vi "CFWSWebClient.vi"(4 "Scan Period":dbl format="%.2f", 5 "Previous Scan Value":dbl format="%.2f", 6 "Present scan array":dbl[](array[numeric]) format="%.2f", 7 "Value to Output":dbl format="%.2f", 8 "Ch Description":T1={"Ch Name"="", "Type"="", "Function"=enum."Analogue Input", "Ch State"=enum."On", "Calibration type"="", "A"=0.0, "B"=0.0, "C"=0.0, "D"=0.0, "Comments"="", "Address"={"Main"=0, "Ch."=0, "Sub"=0, "Port Name"=""}, "String"="", "Duty"=65535} {"Duty" format="%016b"; "D" format="%#_5g"; "C" format="%#_5g"; "B" format="%#_5g"; "A" format="%#_5g"}, 9 "Ch names":string[](array[string])) -> (0 "Scan comment":string, 1 "Output":dbl format="%.3f")   [LabVIEW 2016]
uses:
  ADAM Client/Sub VIs/ADAM Controls/Ch_description_ADAM.ctl
  ADAM Client/Sub VIs/ADAM Controls/Module_type_ADAM.ctl
  ADAM Client/Sub VIs/ADAM Controls/Function_ADAM.ctl
  ADAM Client/Sub VIs/ADAM Controls/Channel_State.ctl
  ADAM Client/Sub VIs/ADAM Controls/Calib_type_ADAM.ctl
  ADAM Client/Sub VIs/ADAM Controls/Address.ctl
  ADAM Client/Sub VIs/ADAM Controls/Remember_value_mode.ctl
panel:
  out "TimeToUpdate?":bool
  in  "stop":bool
  out "Time Of Value (s)":dbl format="%.2f"
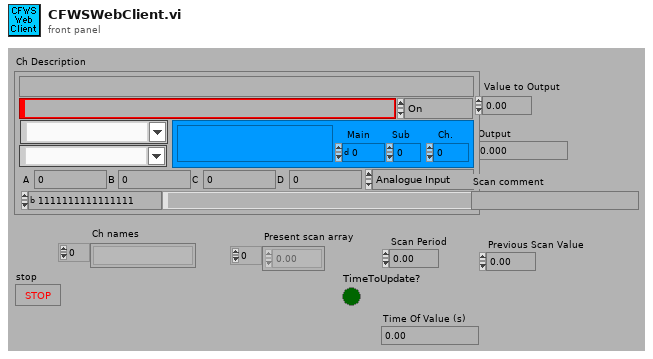
[diagram p1: front panel]
types:
  T1 = typedef "Ch_description_ADAM.ctl" = cluster{"Ch Name":string, "Type":T2, "Function":T3, "Ch State":T4, "Calibration type":T5, "A":dbl, "B":dbl, "C":dbl, "D":dbl, "Comments":string, "Address":T6, "String":string, "Duty":u16}
  T2 = typedef "Module_type_ADAM.ctl" = string
  T3 = typedef "Function_ADAM.ctl" = enum16{"Analogue Input", "Digital Input", "Event counter", "Event rate", "Analogue Output", "Digital Output", "Relay Output"}
  T4 = typedef "Channel_State.ctl" = enum16{"On", "Off", "Always On", "Always Off"}
  T5 = typedef "Calib_type_ADAM.ctl" = string
  T6 = typedef "Address.ctl" = cluster{"Main":i32, "Ch.":i32, "Sub":i32, "Port Name":string}
  T7 = typedef "Remember_value_mode.ctl" = enum16{"Read only", "Read and Write"}
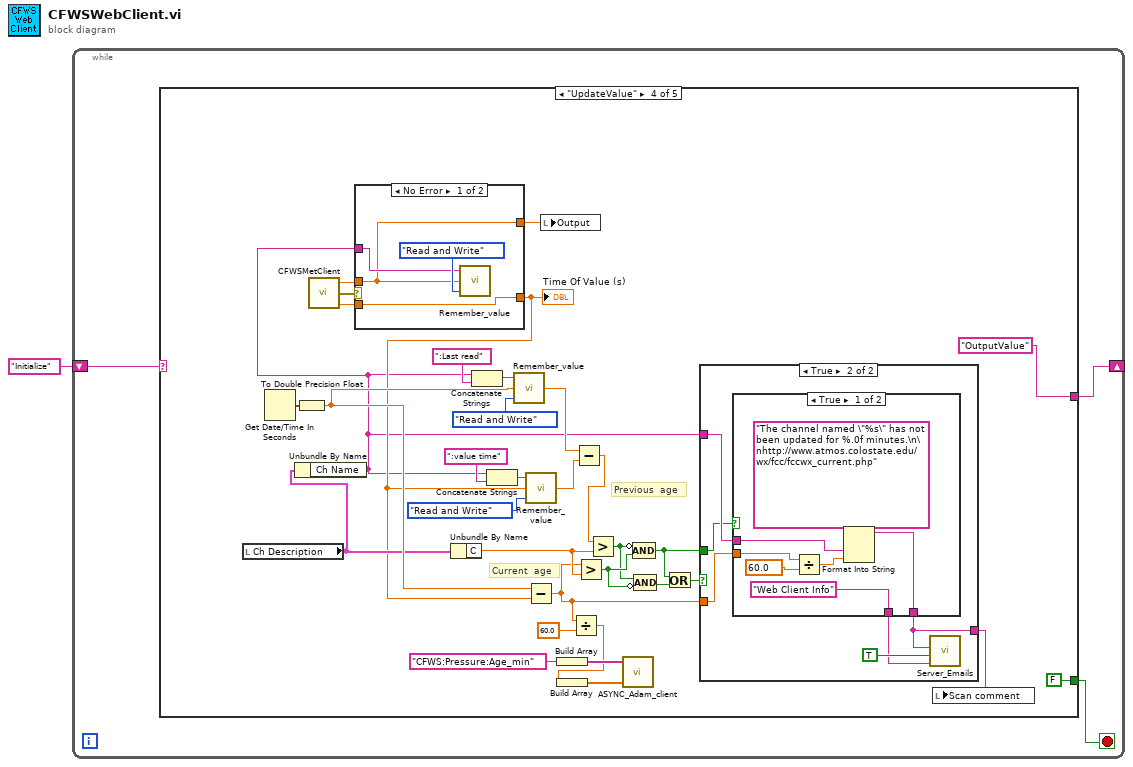
[diagram p0: block diagram]
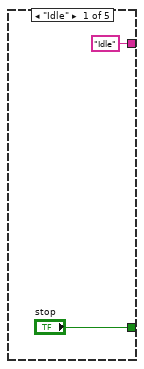
[diagram p2: hidden frame]
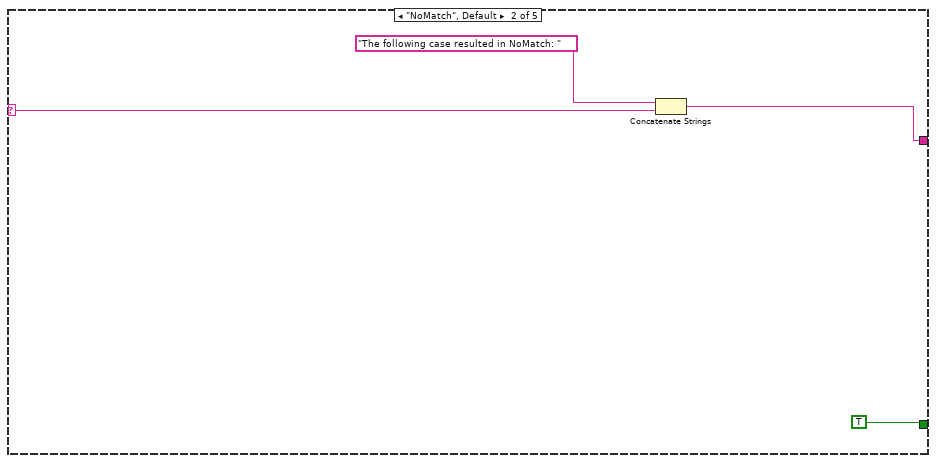
[diagram p3: hidden frame]
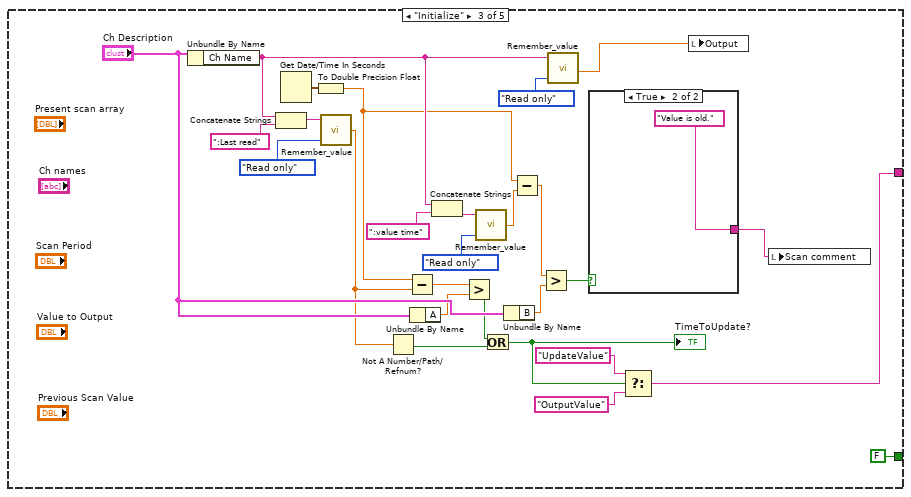
[diagram p4: hidden frame]
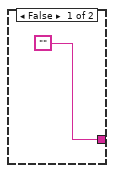
[diagram p5: hidden frame]
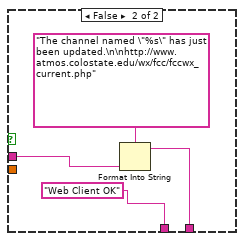
[diagram p7: hidden frame]
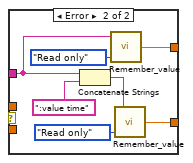
[diagram p8: hidden frame]
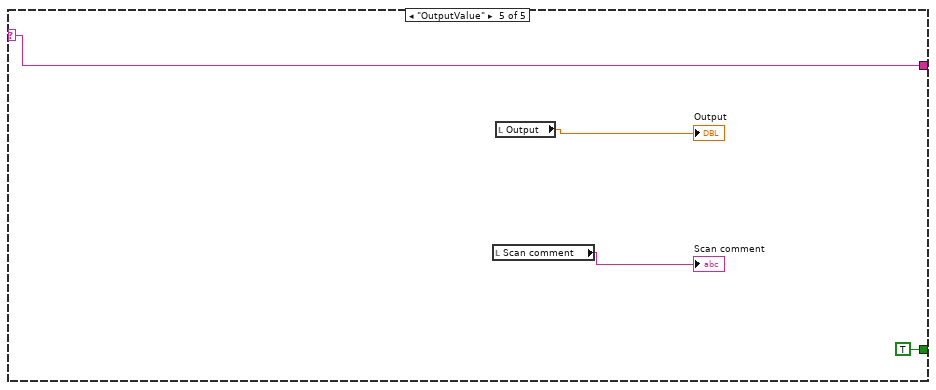
[diagram p9: hidden frame]
diagram:
  n1 = while {
    shift-right: [w3] -> _
    shift-left: "Initialize" -> [w4]
    stop <- w2 stop-if-true
    n2 = case shown="\"UpdateValue\"" w4 {
      selector: w4 -> [_ w8 _ _ w105]
      tunnel: ["Idle" w7 w11 "OutputValue" w105] -> w3
      tunnel: ["stop" TRUE FALSE ("stop") FALSE ("stop") TRUE ("stop")] -> w2
      frame "Idle" {
      }
      frame "NoMatch", Default {
        n3 = Concatenate Strings("The following case resulted in NoMatch: " ("string"), w8) -> (w7:string)
      }
      frame "Initialize" {
        n4 = Unbundle By Name("Ch Description") -> ("Ch Name"=w33:string)
        n5 = Concatenate Strings(w33, ":Last read" ("Substring")) -> (w20:string)
        n6 = Get Date/Time In Seconds() -> (seconds since 1Jan1904=w25:timestamp)
        n7 = To Double Precision Float(number=w25) -> (double precision float=w27:dbl)
        n8 = call "Remember_value.vi"("Mode"=Remember_value_mode."Read only", "Ch name"=w20) -> ("Output Value"=w21:dbl)  [unwired: 1 in]
        n9 = Not A Number/Path/Refnum?(number/path/refnum=w21) -> (NaN/Path/Refnum?=w23:bool)
        n10 = Subtract(x=w27, y=w21) -> (x-y=w17:dbl)
        n11 = Unbundle By Name("Ch Description") -> ("A"=w34:dbl)
        n12 = Concatenate Strings(w33, ":value time" ("Substring")) -> (w31:string)
        n13 = Greater?(x=w17, y=w34) -> (0:w22:bool)
        n14 = call "Remember_value.vi"("Mode"=Remember_value_mode."Read only", "Ch name"=w31) -> ("Output Value"=w26:dbl)  [unwired: 1 in]
        n15 = Or(x=w22, y=w23) -> (x .or. y?=w14:bool)
        "TimeToUpdate?" <- w14
        n16 = Unbundle By Name("Ch Description") -> ("B"=w35:dbl)
        n17 = Subtract(x=w27, y=w26) -> (x-y=w28:dbl)
        n18 = Greater?(x=w28, y=w35) -> (0:w24:bool)
        n19 = call "Remember_value.vi"("Mode"=Remember_value_mode."Read only", "Ch name"=w33) -> ("Output Value"=w16:dbl)  [unwired: 1 in]
        n20 = case shown="True" w24 {
          tunnel: ["" "Value is old." ("Format String")] -> w15
          frame False {
          }
          frame True {
          }
        }
        n21 = Select(t="UpdateValue", s=w14, f="OutputValue") -> (s? t:f=w11:string)
        n22 = local write "Output"(w16) -> ()
        n23 = local write "Scan comment"(w15) -> ()
      }
      frame "UpdateValue" {
        # "Previous  age"
        # "Current  age"
        n24 = local read "Ch Description"() -> (w54:T1)
        n25 = Get Date/Time In Seconds() -> (seconds since 1Jan1904=w63:timestamp)
        n26 = Unbundle By Name(w54) -> ("Ch Name"=w52:string)
        n27 = To Double Precision Float(number=w63) -> (double precision float=w69:dbl)
        n28 = call "CFWSMetClient.vi"() -> ("Time Of Value (s)"=w42:dbl, "error out"=w41:errorcluster, "RawPressure/mBar"=w40:dbl)
        n29 = case shown="No Error" w41 {
          tunnel: [w91 w95] -> w72
          tunnel: [w94 w96] -> w53
          tunnel: w52 -> [w92 w98]
          tunnel: w40 -> [w91 _]
          tunnel: w42 -> [w94 _]
          frame No Error {
            n30 = call "Remember_value.vi"("Mode"=Remember_value_mode."Read and Write", "Input Value"=w91, "Ch name"=w92) -> ()  [unwired: 1 out]
          }
          frame Error {
            n31 = Concatenate Strings(w98, ":value time" ("Substring")) -> (w97:string)
            n32 = call "Remember_value.vi"("Mode"=Remember_value_mode."Read only", "Ch name"=w98) -> ("Output Value"=w95:dbl)  [unwired: 1 in]
            n33 = call "Remember_value.vi"("Mode"=Remember_value_mode."Read only", "Ch name"=w97) -> ("Output Value"=w96:dbl)  [unwired: 1 in]
          }
        }
        "Time Of Value (s)" <- w53
        n34 = Unbundle By Name(w54) -> ("C"=w71:dbl)
        n35 = Concatenate Strings(w52, ":Last read" ("Substring")) -> (w68:string)
        n36 = Concatenate Strings(w52, ":value time" ("Substring")) -> (w57:string)
        n37 = call "Remember_value.vi"("Mode"=Remember_value_mode."Read and Write", "Input Value"=w69, "Ch name"=w68) -> ("Output Value"=w70:dbl)
        n38 = call "Remember_value.vi"("Mode"=Remember_value_mode."Read and Write", "Input Value"=w53, "Ch name"=w57) -> ("Output Value"=w64:dbl)
        n39 = Subtract(x=w69, y=w53) -> (x-y=w45:dbl)
        n40 = local write "Output"(w72) -> ()
        n41 = Build Array("CFWS:Pressure:Age_min") -> (w46:string[])
        n42 = Divide(x=w45, y=60.0) -> (x/y=w43:dbl)
        n43 = Build Array(w43) -> (w47:dbl[])
        n44 = Subtract(x=w70, y=w64) -> (x-y=w65:dbl)
        n45 = Greater?(x=w45, y=w71) -> (0:w59:bool)
        n46 = Greater?(x=w65, y=w71) -> (0:w58:bool)
        n47 = call "ASYNC_Adam_client.vi"("Values"=w47, "Channel Names"=w46) -> ()  [unwired: 1 in, 2 out]
        n48 = Compound Arithmetic op=AND(invert w58, w59) -> (w62:bool)
        n49 = Compound Arithmetic op=AND(w58, invert w59) -> (w60:bool)
        n50 = Or(x=w62, y=w60) -> (x .or. y?=w61:bool)
        n51 = case shown="True" w61 {
          tunnel: w45 -> [_ w79]
          tunnel: w52 -> [_ w78]
          tunnel: w62 -> [_ w77]
          tunnel: ["" w74] -> w51
          frame False {
          }
          frame True {
            n52 = case shown="True" w77 {
              tunnel: w79 -> [w84 _]
              tunnel: w78 -> [w86 w90]
              tunnel: [w81 w88] -> w74
              tunnel: ["Web Client Info" ("Subject") "Web Client OK" ("Subject")] -> w75
              frame True {
                n53 = Divide(x=w84, y=60.0) -> (x/y=w83:dbl)
                n54 = Format Into String(format string="The channel named \"%s\" has not been updated for %.0f minutes.\n\nhttp://www.atmos.colostate.edu/wx/fcc/fccwx_current.php" ("Format String"), w86, w83) -> (resulting string=w81:string)  [unwired: 2 in, 1 out]
              }
              frame False {
                n55 = Format Into String(format string="The channel named \"%s\" has just been updated.\n\nhttp://www.atmos.colostate.edu/wx/fcc/fccwx_current.php" ("Format String"), w90) -> (resulting string=w88:string)  [unwired: 2 in, 1 out]
              }
            }
            n56 = call "Server_Emails.vi"("Message"=w74, "Contact All clients?"=TRUE, "Subject"=w75) -> ()  [unwired: 2 in, 3 out]
          }
        }
        n57 = local write "Scan comment"(w51) -> ()
      }
      frame "OutputValue" {
        n58 = local read "Scan comment"() -> (→"Scan comment":string)
        n59 = local read "Output"() -> (→"Output":dbl)
      }
    }
  }
